vi "remove_multiple_function_variables.vi"(1 "function\nvariables":string[](array[string])) -> (0 "unique\nfunction\nvariables":string[](array[string]))   [LabVIEW 2010]
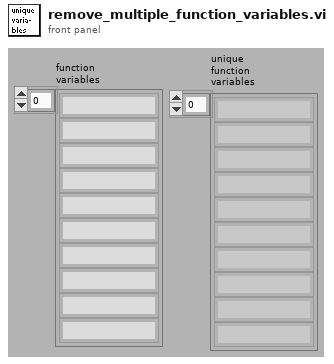
[diagram p1: front panel]
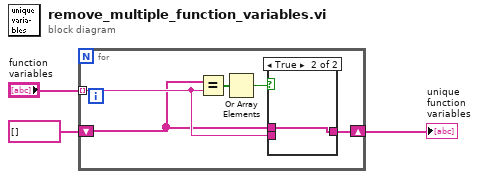
[diagram p0: block diagram]
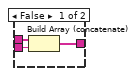
[diagram p2: hidden frame]
diagram:
  n1 = for {
    tunnel: "function\nvariables" -> [w5] mode=indexing
    shift-right: [w6] -> w1
    shift-left: string[] [] -> [w4]
    n2 = Equal?(x=w4, y=w5) -> (x = y?=w8:bool[])
    n3 = Or Array Elements(Boolean array=w8) -> (logical OR=w7:bool)
    n4 = case shown="True" w7 {
      tunnel: w5 -> [w11 _]
      tunnel: [w10 w12] -> w6
      tunnel: w4 -> [w9 w12]
      frame False {
        n5 = Build Array (concatenate)(w9, w11) -> (w10:string[])
      }
      frame True {
      }
    }
  }
  "unique\nfunction\nvariables" <- w1
